vi "Set Magnet Vector.vi"(8 "error in (no error)":errorcluster, 9 "Target Rate Limit (T/min)":dbl, 10 "Target Field (T)":dbl[](array[numeric]), 11 "Instrument.VRM in":refnum<class "Instrument.OxfordVRM.lvclass">) -> (0 "error out":errorcluster, 3 "Instrument.VRM out":refnum<class "Instrument.OxfordVRM.lvclass">)   [LabVIEW 2019, in "Instrument.OxfordVRM.lvclass"]
uses:
  Instrument.OxfordVRM.lvclass
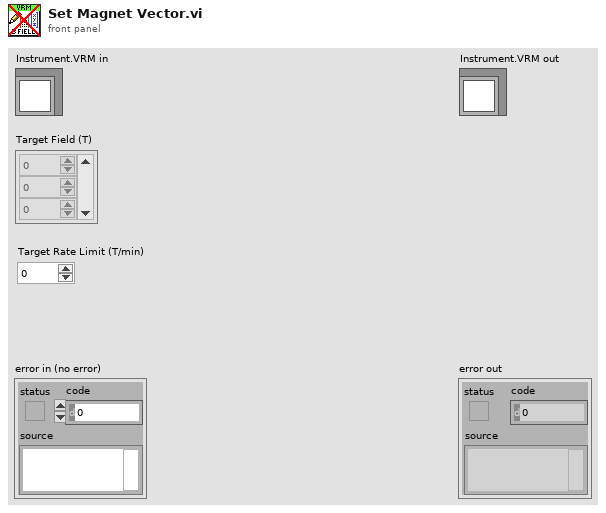
[diagram p1: front panel]
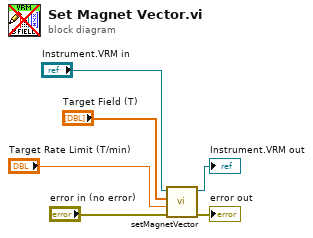
[diagram p0: block diagram]
diagram:
  n1 = call-dynamic "setMagnetVector.vi"("error in (no error)"="error in (no error)", "Target Rate Limit (T/min)"="Target Rate Limit (T/min)", "Target Field (T)"="Target Field (T)", "Instrument.VRM in"="Instrument.VRM in") -> ("error out"=→"error out":errorcluster, "Instrument.VRM out"=→"Instrument.VRM out":refnum<class "Instrument.OxfordVRM.lvclass">)  [unwired: 6 in]
